vi "Requests.vi"(8 "error in (no error)":errorcluster, 9 "write enable":bool=TRUE, 11 "ICPCON ET7028 in":refnum<class "ICPCON ET-7028.lvclass">) -> (0 "error out":errorcluster, 3 "ICPCON ET7028 out":refnum<class "ICPCON ET-7028.lvclass">)   [LabVIEW 2021, in "ICPCON ET-7028.lvclass"]
uses:
  ICPCON ET-7028.lvclass
  D:/my_projects/projects/Algorithms/Labview/21/Master CR/Master CR.lvclass
  D:/my_projects/projects/Algorithms/Labview/21/Master CR/Devices/ET7000/TCP/TCP.lvclass
  Master CR.lvclass/Master CR.ctl
  Modbus_v121c/Modbus Data Unit/Modbus Data Unit.lvclass/Modbus Data Unit.ctl
  Modbus_v121c/Network Protocol/Network Master/Network Master.lvclass/Network Master.ctl
  Modbus_v121c/Master Function Definition/Write Multiple Registers Request.vi
  Modbus_v121c/Master Function Definition/Function data mismatch error.vi
  Modbus_v121c/Master Function Definition/Write Multiple Registers Response.vi
  Modbus_v121c/Network Protocol/Network Master/Read write Master.vi
  Modbus_v121c/Master Function Definition/Read Holding Registers Request.vi
  Modbus_v121c/Master Function Definition/Read Holding Registers Response.vi
  Network Protocol/Read Network Protocol.vi
  Modbus_v121c/Modbus Data Unit/Construct PDU.vi
  Modbus_v121c/Utility/U16s to Bytes.vi
  Modbus_v121c/Master Function Definition/Function code mismatch error.vi
  Modbus_v121c/Data Model/Error Generator.vi
  Modbus_v121c/Modbus Data Unit/Deconstruct PDU.vi
  Modbus_v121c/Utility/Bytes to U16s.vi
  TCP/TCP.lvclass
  Modbus_v121c/Network Protocol/Network Master/Network Master.lvclass
  Modbus_v121c/Modbus Data Unit/Modbus Data Unit.lvclass
  Modbus_v121c/Data Model/Device Data Model.lvclass
  Modbus_v121c/Transmission Data Unit/Transmission Data Unit.lvclass
  Master CR.lvclass
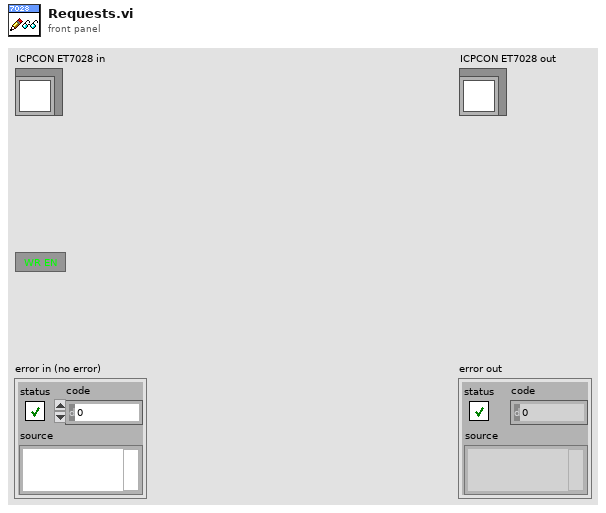
[diagram p1: front panel]
types:
  T1 = typedef "Device Data Model.lvclass/N channel.ctl" = cluster{"N DI channel":i32, "N DO channel":i32, "N AI channel":i32, "N AO channel":i32}
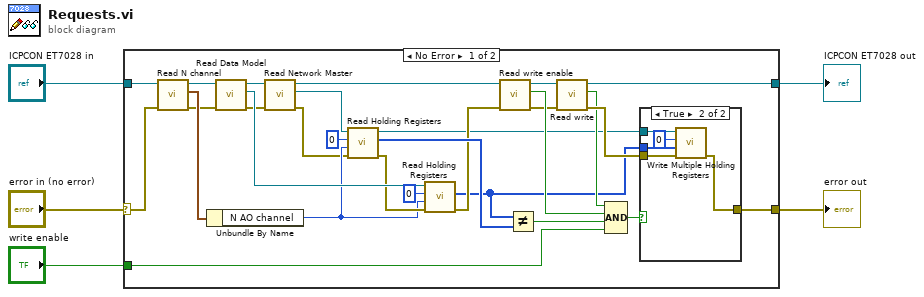
[diagram p0: block diagram]
diagram:
  n1 = case shown="No Error" "error in (no error)" {
    selector: "error in (no error)" -> [w29 w42]
    tunnel: [w33 w42] -> w3
    tunnel: [w11 w41] -> w4
    tunnel: "ICPCON ET7028 in" -> [w31 w41]
    tunnel: "write enable" -> [w25 _]
    frame No Error {
      n2 = call "Read N channel.vi"("error in (no error)"=w29, "Master CR in"=w31) -> ("error out"=w28:errorcluster, "N channel"=w32:T1, "Master CR out"=w30:refnum<class "ICPCON ET-7028.lvclass">)  [unwired: 7 in]
      n3 = Unbundle By Name(w32) -> ("N AO channel"=w14:i32)
      n4 = call "Read Data Model.vi"("error in (no error)"=w28, "Master CR in"=w30) -> ("error out"=w10:errorcluster, "Data Model"=w19:refnum<class "Device Data Model.lvclass">, "Master CR out"=w9:refnum<class "ICPCON ET-7028.lvclass">)  [unwired: 7 in]
      n5 = call "Read Network Master.vi"("error in (no error)"=w10, "TCP in"=w9) -> ("error out"=w7:errorcluster, "Network Master"=w6:refnum<class "Network Master.lvclass">, "TCP out"=w8:refnum<class "ICPCON ET-7028.lvclass">)  [unwired: 7 in]
      n6 = call "Read Holding Registers.vi"("error in (no error)"=w7, "number of holding registers"=w14, "starting address"=u16 0, "Modbus master in"=w6) -> ("error out"=w15:errorcluster, "register values"=w17:u16[], "Modbus master out"=w12:refnum<class "Network Master.lvclass">)  [unwired: 5 in]
      n7 = call-dynamic "Read Holding Registers.vi"("error in"=w15, "number of registers"=w14, "starting address"=u16 0, "device data model in"=w19) -> ("error out"=w16:errorcluster, "data"=w13:u16[])  [unwired: 5 in, 1 out]
      n8 = call "Read write enable.vi"("error in (no error)"=w16, "Master CR in"=w8) -> ("error out"=w23:errorcluster, "write enable"=w26:bool, "Master CR out"=w24:refnum<class "ICPCON ET-7028.lvclass">)  [unwired: 7 in]
      n9 = Not Equal?(x=w13, y=w17) -> (x != y?=w27:bool)
      n10 = call "Read write.vi"("error in (no error)"=w23, "Master CR in"=w24) -> ("error out"=w22:errorcluster, "Write"=w21:bool, "Master CR out"=w11:refnum<class "ICPCON ET-7028.lvclass">)  [unwired: 7 in]
      n11 = Compound Arithmetic op=AND(w21, w26, w27, w25) -> (w34:bool)
      n12 = case shown="True" w34 {
        tunnel: w22 -> [w35 w38]
        tunnel: [w35 w36] -> w33
        tunnel: w13 -> [_ w37]
        tunnel: w12 -> [_ w39]
        frame False {
        }
        frame True {
          n13 = call "Write Multiple Holding Registers.vi"("error in (no error)"=w38, "holding register values"=w37, "starting address"=u16 0, "Modbus master in"=w39) -> ("error out"=w36:errorcluster)  [unwired: 6 in, 1 out]
        }
      }
    }
    frame Error {
    }
  }
  "error out" <- w3
  "ICPCON ET7028 out" <- w4
